vi "Lucky Draw.vi"() -> ()   [LabVIEW 2018]
uses:
  <vilib>/Utility/file.llb/Read Delimited Spreadsheet (string).vi
  <vilib>/Utility/file.llb/Write Delimited Spreadsheet (string).vi
panel:
  out "Listbox":i32(listbox)
  in  "Begin Draw !!!":bool
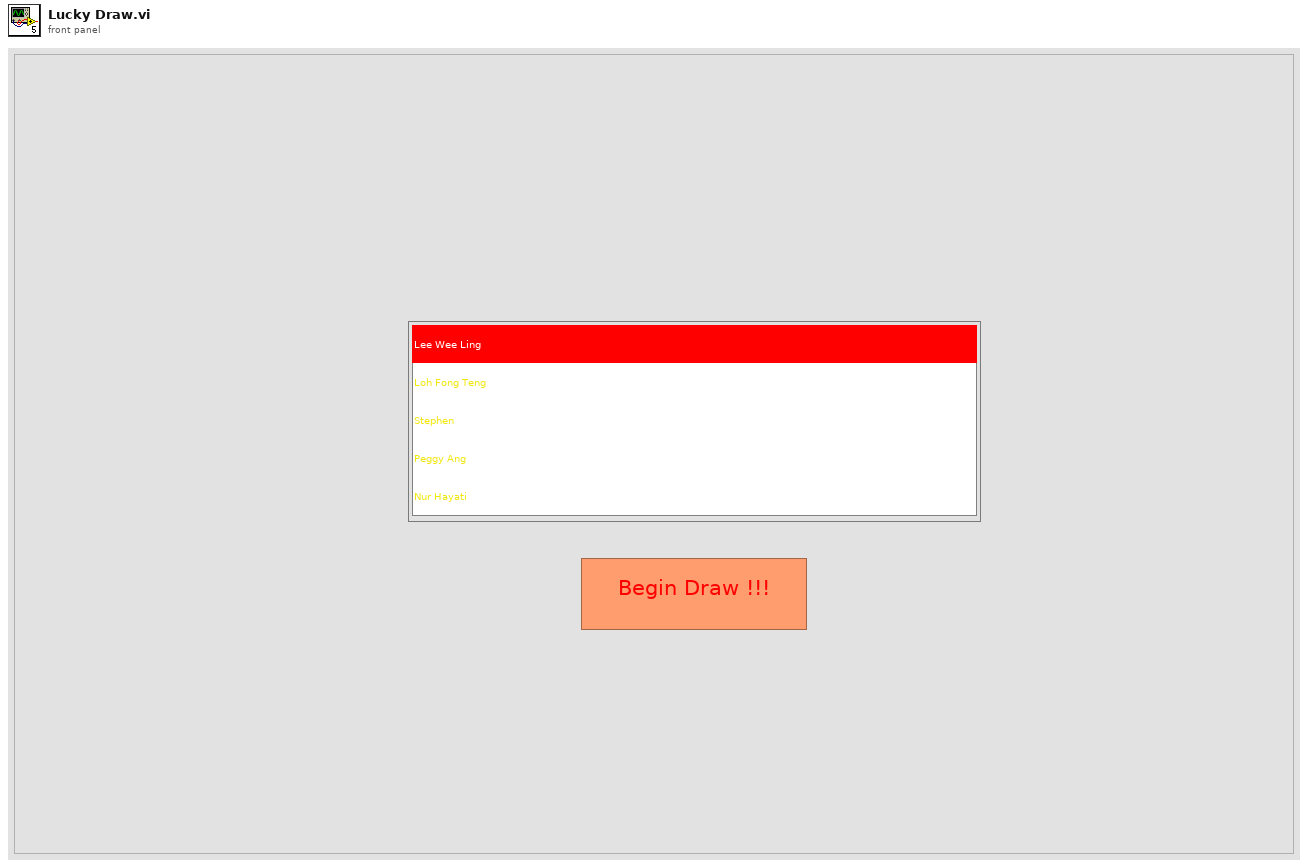
[diagram p1: front panel]
types:
  T1 = enum8{"Enabled", "Disabled", "Disabled and Grayed Out"}
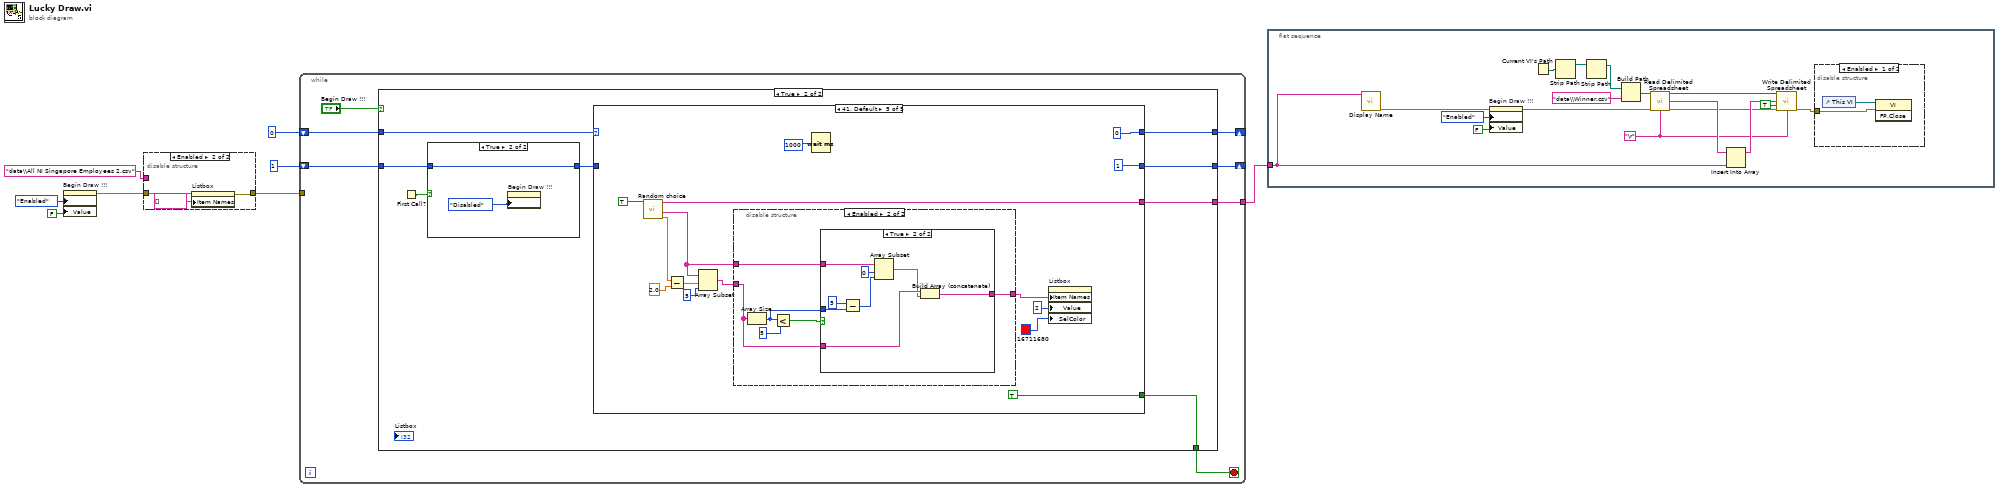
[diagram p0: block diagram]
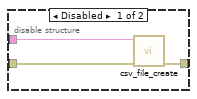
[diagram p2: hidden frame]
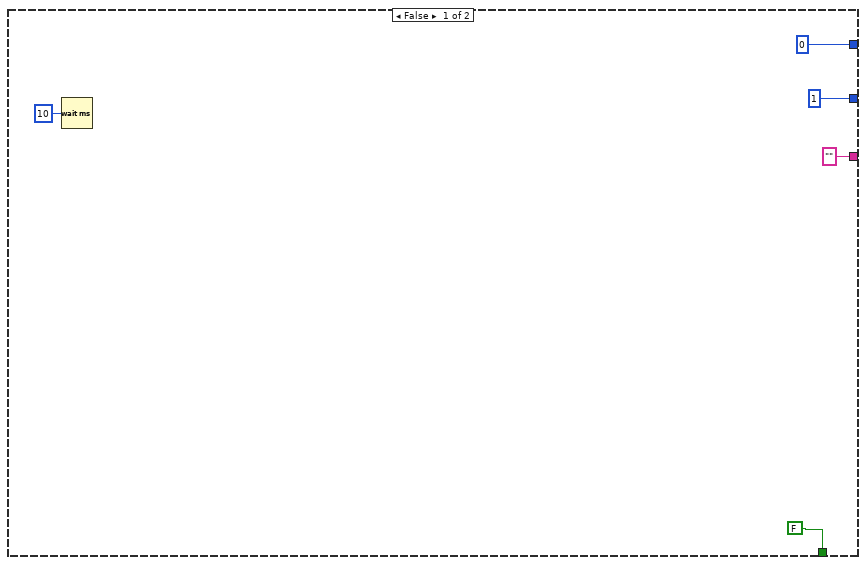
[diagram p4: hidden frame]
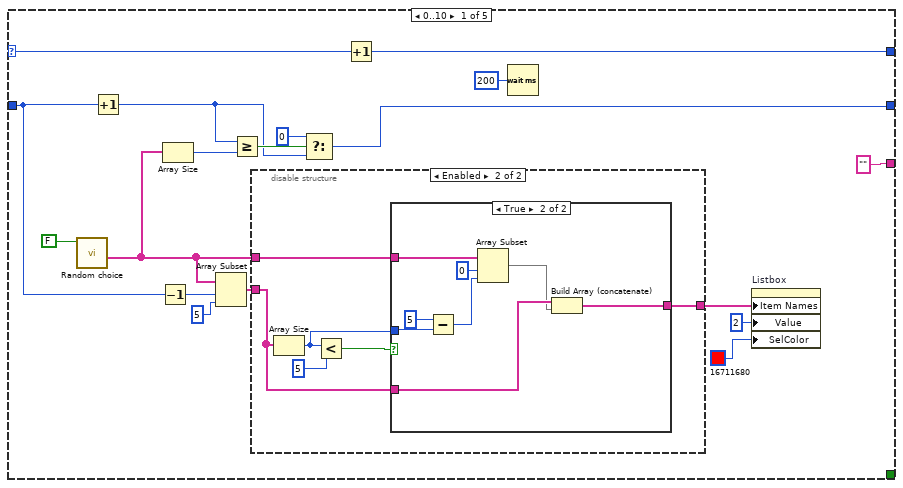
[diagram p6: hidden frame]
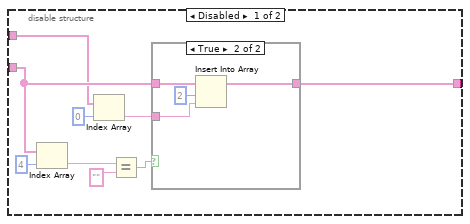
[diagram p7: hidden frame]
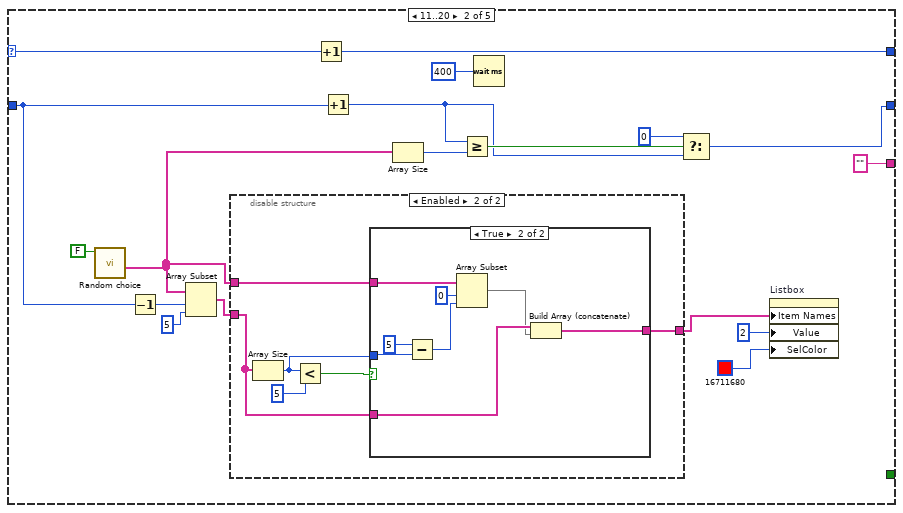
[diagram p10: hidden frame]
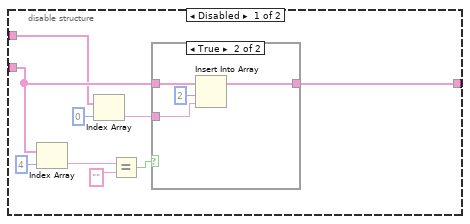
[diagram p11: hidden frame]
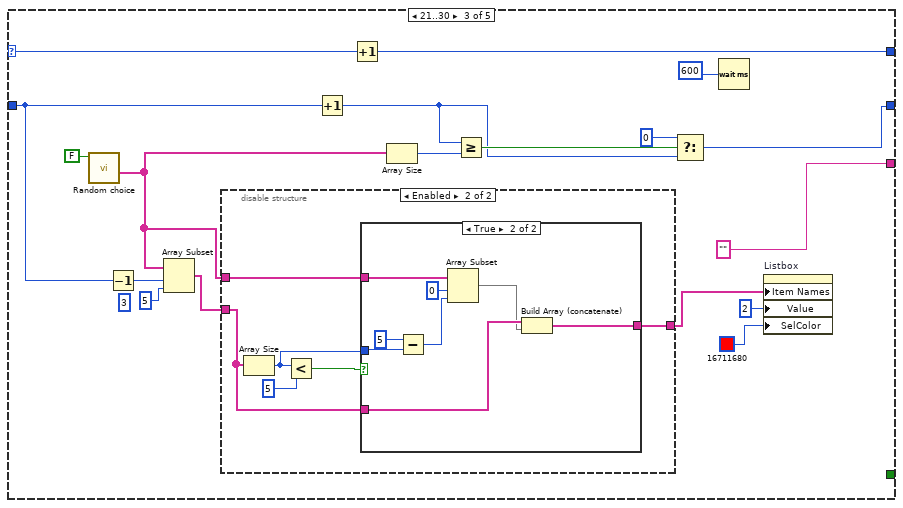
[diagram p14: hidden frame]
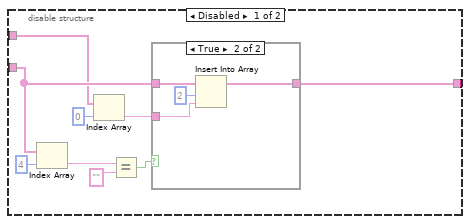
[diagram p15: hidden frame]
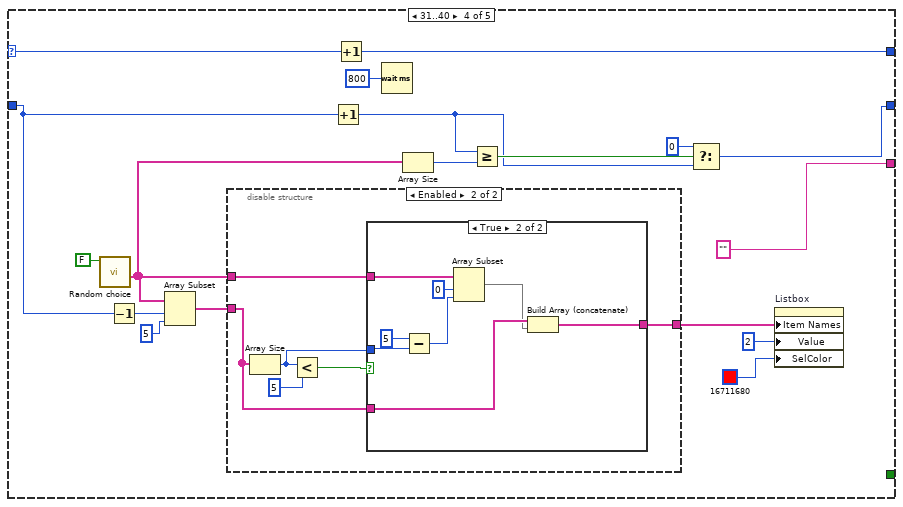
[diagram p18: hidden frame]
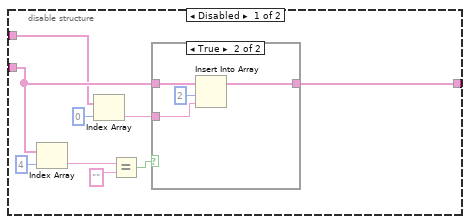
[diagram p19: hidden frame]
diagram:
  n1 = property on="Begin Draw !!!" class="Bool (strict)"("DisabledEnum"=T1."Enabled" ("Disabled"), "Value"=FALSE ("Begin Draw !!!")) -> (error out=w3:errorcluster)  [unwired: 2 in, 1 out]
  n2 = disable-structure shown="Enabled" {
    disable-tunnel: w3 -> [w11 w14]
    disable-tunnel: [w10 w13] -> w2
    disable-tunnel: "data\\All NI Singapore Employees 2.csv" ("name or relative path") -> [w9 _]
    frame Disabled {
      n3 = call "csv_file_create.vi"("error in (no error)"=w11, "name or relative path"=w9) -> ("error out"=w10:errorcluster)  [unwired: 8 in, 1 out]
    }
    frame Enabled {
      n4 = property on="Listbox" class="LstBox (strict)"(error in=w14, "Item Names"=string[] []) -> (error out=w13:errorcluster)  [unwired: 1 in, 1 out]
    }
  }
  n5 = while {
    shift-right: [w18] -> _
    shift-left: u32 0 ("x") -> [w19]
    shift-right: [w16] -> _
    shift-left: u32 1 ("x") -> [w17]
    tunnel: [w15] -> w6
    tunnel: w2 -> [_]
    stop <- w21 stop-if-true
    n6 = case shown="True" "Begin Draw !!!" {
      tunnel: [FALSE ("Boolean") w32] -> w21
      tunnel: w19 -> [_ w33]
      tunnel: [u32 0 ("x") w34] -> w18
      tunnel: w17 -> [_ w28]
      tunnel: [u32 1 ("t") w31] -> w16
      tunnel: ["" ("Choice") w30] -> w15
      frame False {
        n7 = Wait (ms)(milliseconds to wait=u32 10) -> ()  [unwired: 1 out]
      }
      frame True {
        n8 = First Call?() -> (First Call?: T/F=w29:bool)
        n9 = case shown="True" w29 {
          tunnel: w28 -> [w35 w36]
          tunnel: [w35 w36] -> w27
          frame False {
          }
          frame True {
            n10 = property on="Begin Draw !!!" class="Bool (strict)"("DisabledEnum"=T1."Disabled" ("Disabled")) -> ()  [unwired: 2 in, 2 out]
          }
        }
        n11 = case shown="41, Default" w33 {
          selector: w33 -> [w55 w102 w149 w196 _]
          tunnel: [w54 w101 w148 w195 u32 0] -> w34
          tunnel: [_ _ _ _ TRUE ("Boolean")] -> w32
          tunnel: w27 -> [w45 w90 w136 w183 _]
          tunnel: [w39 w89 w137 w184 u32 1] -> w31
          tunnel: ["" ("Choice") "" ("Choice") "" ("Choice") "" ("Choice") w230] -> w30
          frame 0..10 {
            n12 = call "Random choice.vi"("Selection Made"=FALSE) -> ("shuffled names"=w44:string[])  [unwired: 8 in, 2 out]
            n13 = Increment(x=w45) -> (x+1=w40:u32)
            n14 = Decrement(x=w45) -> (x-1=w53:u32)
            n15 = Array Size(array=w44) -> (size(s)=w43:i32)
            n16 = Array Subset(array=w44, index=w53, length=5) -> (w50:string[])
            n17 = Greater Or Equal?(x=w40, y=w43) -> (x >= y?=w42:bool)
            n18 = disable-structure shown="Enabled" {
              disable-tunnel: w50 -> [w61 w71]
              disable-tunnel: [w57 w70] -> w49
              disable-tunnel: w44 -> [w56 w72]
              frame Disabled {
                n19 = Index Array(array=w61, index=4) -> (element=w63:string)
                n20 = Index Array(array=w56, index=0) -> (element=w59:string)
                n21 = Equal?(x=w63, y="") -> (x = y?=w58:bool)
                n22 = case shown="True" w58 {
                  tunnel: w61 -> [w65 w69]
                  tunnel: w59 -> [_ w67]
                  tunnel: [w65 w66] -> w57
                  frame False {
                  }
                  frame True {
                    n23 = Insert Into Array(array=w69, index=2, new element=w67) -> (w66:string[])
                  }
                }
              }
              frame Enabled {
                n24 = Array Size(array=w71) -> (size(s)=w73:i32)
                n25 = Less?(x=w73, y=5) -> (x < y?=w74:bool)
                n26 = case shown="True" w74 {
                  tunnel: w73 -> [_ w84]
                  tunnel: w72 -> [_ w82]
                  tunnel: w71 -> [w76 w79]
                  tunnel: [w76 w77] -> w70
                  frame False {
                  }
                  frame True {
                    n27 = Subtract(x=5, y=w84) -> (x-y=w80:i32)
                    n28 = Array Subset(array=w82, index=0, length=w80) -> (w78:string[])
                    n29 = Build Array (concatenate)(w79, w78) -> (w77:string[])
                  }
                }
              }
            }
            n30 = Select(t=u32 0, s=w42, f=w40) -> (s? t:f=w39:u32)
            n31 = Increment(x=w55) -> (x+1=w54:u32)
            n32 = Wait (ms)(milliseconds to wait=u32 200) -> ()  [unwired: 1 out]
            n33 = property on="Listbox" class="LstBox (strict)"("Item Names"=w49, "Value"=2 ("Active Row:Active Row Number"), "SelColor"=u32 16711680) -> ()  [unwired: 2 in, 2 out]
          }
          frame 11..20 {
            n34 = call "Random choice.vi"("Selection Made"=FALSE) -> ("shuffled names"=w86:string[])  [unwired: 8 in, 2 out]
            n35 = Decrement(x=w90) -> (x-1=w100:u32)
            n36 = Array Subset(array=w86, index=w100, length=5) -> (w87:string[])
            n37 = disable-structure shown="Enabled" {
              disable-tunnel: w87 -> [w108 w118]
              disable-tunnel: [w104 w117] -> w85
              disable-tunnel: w86 -> [w103 w119]
              frame Disabled {
                n38 = Index Array(array=w108, index=4) -> (element=w110:string)
                n39 = Index Array(array=w103, index=0) -> (element=w106:string)
                n40 = Equal?(x=w110, y="") -> (x = y?=w105:bool)
                n41 = case shown="True" w105 {
                  tunnel: w108 -> [w112 w116]
                  tunnel: w106 -> [_ w114]
                  tunnel: [w112 w113] -> w104
                  frame False {
                  }
                  frame True {
                    n42 = Insert Into Array(array=w116, index=2, new element=w114) -> (w113:string[])
                  }
                }
              }
              frame Enabled {
                n43 = Array Size(array=w118) -> (size(s)=w120:i32)
                n44 = Less?(x=w120, y=5) -> (x < y?=w121:bool)
                n45 = case shown="True" w121 {
                  tunnel: w120 -> [_ w131]
                  tunnel: w119 -> [_ w129]
                  tunnel: w118 -> [w123 w126]
                  tunnel: [w123 w124] -> w117
                  frame False {
                  }
                  frame True {
                    n46 = Subtract(x=5, y=w131) -> (x-y=w127:i32)
                    n47 = Array Subset(array=w129, index=0, length=w127) -> (w125:string[])
                    n48 = Build Array (concatenate)(w126, w125) -> (w124:string[])
                  }
                }
              }
            }
            n49 = Increment(x=w102) -> (x+1=w101:u32)
            n50 = Increment(x=w90) -> (x+1=w92:u32)
            n51 = Array Size(array=w86) -> (size(s)=w94:i32)
            n52 = Greater Or Equal?(x=w92, y=w94) -> (x >= y?=w93:bool)
            n53 = Wait (ms)(milliseconds to wait=u32 400) -> ()  [unwired: 1 out]
            n54 = Select(t=u32 0, s=w93, f=w92) -> (s? t:f=w89:u32)
            n55 = property on="Listbox" class="LstBox (strict)"("Item Names"=w85, "Value"=2 ("Active Row:Active Row Number"), "SelColor"=u32 16711680) -> ()  [unwired: 2 in, 2 out]
          }
          frame 21..30 {
            (unwired) 3 ("length")
            n56 = call "Random choice.vi"("Selection Made"=FALSE) -> ("shuffled names"=w133:string[])  [unwired: 8 in, 2 out]
            n57 = Decrement(x=w136) -> (x-1=w147:u32)
            n58 = Array Subset(array=w133, index=w147, length=5) -> (w134:string[])
            n59 = disable-structure shown="Enabled" {
              disable-tunnel: w134 -> [w155 w165]
              disable-tunnel: [w151 w164] -> w132
              disable-tunnel: w133 -> [w150 w166]
              frame Disabled {
                n60 = Index Array(array=w155, index=4) -> (element=w157:string)
                n61 = Index Array(array=w150, index=0) -> (element=w153:string)
                n62 = Equal?(x=w157, y="") -> (x = y?=w152:bool)
                n63 = case shown="True" w152 {
                  tunnel: w155 -> [w159 w163]
                  tunnel: w153 -> [_ w161]
                  tunnel: [w159 w160] -> w151
                  frame False {
                  }
                  frame True {
                    n64 = Insert Into Array(array=w163, index=2, new element=w161) -> (w160:string[])
                  }
                }
              }
              frame Enabled {
                n65 = Array Size(array=w165) -> (size(s)=w167:i32)
                n66 = Less?(x=w167, y=5) -> (x < y?=w168:bool)
                n67 = case shown="True" w168 {
                  tunnel: w167 -> [_ w178]
                  tunnel: w166 -> [_ w176]
                  tunnel: w165 -> [w170 w173]
                  tunnel: [w170 w171] -> w164
                  frame False {
                  }
                  frame True {
                    n68 = Subtract(x=5, y=w178) -> (x-y=w174:i32)
                    n69 = Array Subset(array=w176, index=0, length=w174) -> (w172:string[])
                    n70 = Build Array (concatenate)(w173, w172) -> (w171:string[])
                  }
                }
              }
            }
            n71 = Increment(x=w136) -> (x+1=w139:u32)
            n72 = Increment(x=w149) -> (x+1=w148:u32)
            n73 = Array Size(array=w133) -> (size(s)=w141:i32)
            n74 = Greater Or Equal?(x=w139, y=w141) -> (x >= y?=w140:bool)
            n75 = Select(t=u32 0, s=w140, f=w139) -> (s? t:f=w137:u32)
            n76 = Wait (ms)(milliseconds to wait=u32 600) -> ()  [unwired: 1 out]
            n77 = property on="Listbox" class="LstBox (strict)"("Item Names"=w132, "Value"=2 ("Active Row:Active Row Number"), "SelColor"=u32 16711680) -> ()  [unwired: 2 in, 2 out]
          }
          frame 31..40 {
            n78 = call "Random choice.vi"("Selection Made"=FALSE) -> ("shuffled names"=w180:string[])  [unwired: 8 in, 2 out]
            n79 = Decrement(x=w183) -> (x-1=w194:u32)
            n80 = Array Subset(array=w180, index=w194, length=5) -> (w181:string[])
            n81 = disable-structure shown="Enabled" {
              disable-tunnel: w181 -> [w202 w212]
              disable-tunnel: [w198 w211] -> w179
              disable-tunnel: w180 -> [w197 w213]
              frame Disabled {
                n82 = Index Array(array=w202, index=4) -> (element=w204:string)
                n83 = Index Array(array=w197, index=0) -> (element=w200:string)
                n84 = Equal?(x=w204, y="") -> (x = y?=w199:bool)
                n85 = case shown="True" w199 {
                  tunnel: w202 -> [w206 w210]
                  tunnel: w200 -> [_ w208]
                  tunnel: [w206 w207] -> w198
                  frame False {
                  }
                  frame True {
                    n86 = Insert Into Array(array=w210, index=2, new element=w208) -> (w207:string[])
                  }
                }
              }
              frame Enabled {
                n87 = Array Size(array=w212) -> (size(s)=w214:i32)
                n88 = Less?(x=w214, y=5) -> (x < y?=w215:bool)
                n89 = case shown="True" w215 {
                  tunnel: w214 -> [_ w225]
                  tunnel: w213 -> [_ w223]
                  tunnel: w212 -> [w217 w220]
                  tunnel: [w217 w218] -> w211
                  frame False {
                  }
                  frame True {
                    n90 = Subtract(x=5, y=w225) -> (x-y=w221:i32)
                    n91 = Array Subset(array=w223, index=0, length=w221) -> (w219:string[])
                    n92 = Build Array (concatenate)(w220, w219) -> (w218:string[])
                  }
                }
              }
            }
            n93 = Increment(x=w183) -> (x+1=w186:u32)
            n94 = Increment(x=w196) -> (x+1=w195:u32)
            n95 = Wait (ms)(milliseconds to wait=u32 800) -> ()  [unwired: 1 out]
            n96 = Array Size(array=w180) -> (size(s)=w188:i32)
            n97 = Greater Or Equal?(x=w186, y=w188) -> (x >= y?=w187:bool)
            n98 = Select(t=u32 0, s=w187, f=w186) -> (s? t:f=w184:u32)
            n99 = property on="Listbox" class="LstBox (strict)"("Item Names"=w179, "Value"=2 ("Active Row:Active Row Number"), "SelColor"=u32 16711680) -> ()  [unwired: 2 in, 2 out]
          }
          frame 41, Default {
            n100 = call "Random choice.vi"("Selection Made"=TRUE) -> ("Number Choice"=w240:dbl, "shuffled names"=w229:string[], "Choice"=w230:string)  [unwired: 8 in]
            n101 = Subtract(x=w240, y=2.0 ("x")) -> (x-y=w239:dbl)
            n102 = Array Subset(array=w229, index=w239, length=5) -> (w228:string[])
            n103 = disable-structure shown="Enabled" {
              disable-tunnel: w228 -> [w246 w256]
              disable-tunnel: [w242 w255] -> w227
              disable-tunnel: w229 -> [w241 w257]
              frame Disabled {
                n104 = Index Array(array=w246, index=4) -> (element=w248:string)
                n105 = Index Array(array=w241, index=0) -> (element=w244:string)
                n106 = Equal?(x=w248, y="") -> (x = y?=w243:bool)
                n107 = case shown="True" w243 {
                  tunnel: w246 -> [w250 w254]
                  tunnel: w244 -> [_ w252]
                  tunnel: [w250 w251] -> w242
                  frame False {
                  }
                  frame True {
                    n108 = Insert Into Array(array=w254, index=2, new element=w252) -> (w251:string[])
                  }
                }
              }
              frame Enabled {
                n109 = Array Size(array=w256) -> (size(s)=w258:i32)
                n110 = Less?(x=w258, y=5) -> (x < y?=w259:bool)
                n111 = case shown="True" w259 {
                  tunnel: w258 -> [_ w269]
                  tunnel: w257 -> [_ w267]
                  tunnel: w256 -> [w261 w264]
                  tunnel: [w261 w262] -> w255
                  frame False {
                  }
                  frame True {
                    n112 = Subtract(x=5, y=w269) -> (x-y=w265:i32)
                    n113 = Array Subset(array=w267, index=0, length=w265) -> (w263:string[])
                    n114 = Build Array (concatenate)(w264, w263) -> (w262:string[])
                  }
                }
              }
            }
            n115 = Wait (ms)(milliseconds to wait=u32 1000) -> ()  [unwired: 1 out]
            n116 = property on="Listbox" class="LstBox (strict)"("Item Names"=w227, "Value"=2 ("Active Row:Active Row Number"), "SelColor"=u32 16711680) -> ()  [unwired: 2 in, 2 out]
          }
        }
      }
    }
  }
  n117 = flat-sequence {
    tunnel: w6 -> [w271]
    frame #0 {
      w274 = "\r"
      n118 = call "Display Name.vi"("Name In"=w271) -> ("error out"=w270:errorcluster)  [unwired: 10 in]
      n119 = property on="Begin Draw !!!" class="Bool (strict)"(error in=w270, "DisabledEnum"=T1."Enabled" ("Disabled"), "Value"=FALSE ("Begin Draw !!!")) -> (error out=w279:errorcluster)  [unwired: 1 in, 1 out]
      n120 = Current VI's Path() -> (path=w282:path)
      n121 = Strip Path(path=w282) -> (stripped path=w283:path)  [unwired: 1 out]
      n122 = Strip Path(path=w283) -> (stripped path=w284:path)  [unwired: 1 out]
      n123 = Build Path(base path=w284, name or relative path="data\\Winner.csv") -> (appended path=w280:path)
      n124 = call-poly <vilib>:"Read Delimited Spreadsheet.vi"("file path (dialog if empty)"=w280, "error in (no error)"=w279, "delimiter (\\t)"=w274) -> ("new file path (Not A Path if cancelled)"=w277:path, "first row"=w278:string[], "error out"=w275:errorcluster)  [unwired: 7 in, 3 out]
      n125 = Insert Into Array(array=w278, new element=w271) -> (w276:string[])  [unwired: 1 in]
      n126 = call-poly <vilib>:"Write Delimited Spreadsheet.vi"("file path (dialog if empty)"=w277, "1D data"=w276, "append to file? (new file:F)"=TRUE, "error in (no error)"=w275, "delimiter (\\t)"=w274) -> ("error out"=w272:errorcluster)  [unwired: 9 in, 1 out]
      n127 = disable-structure shown="Enabled" {
        disable-tunnel: w272 -> [w287 _]
        frame Enabled {
          n128 = control-ref of="This VI"() -> (w288:refnum<vi>)
          n129 = invoke class="VI" method="FP.Close"(reference=w288, error in=w287) -> ()  [unwired: 1 in, 3 out]
        }
        frame Disabled {
        }
      }
    }
  }
